vi "GetFileStringBmp.vi"(7 "Color Palette":T1[](array[typedef]), 8 "error in":errorcluster, 9 "Base64 Encoded":bool, 10 "Compress":bool, 11 "Image Reference In":T2) -> (0 "error out":errorcluster, 2 "FileString":string, 3 "Image Reference Out":T2)   [LabVIEW 2020, in "OpenLvVision_Image.lvlib" / "File.lvlib"]
doc: "Returns the entire image content encoded as a string representing an image file, suitable for saving or transferring over the network."
uses:
  File.lvlib
  Management/TypeDef/Image.ctl
  TypeDef/ColorPaletteValue.ctl
  Management/Management.lvlib
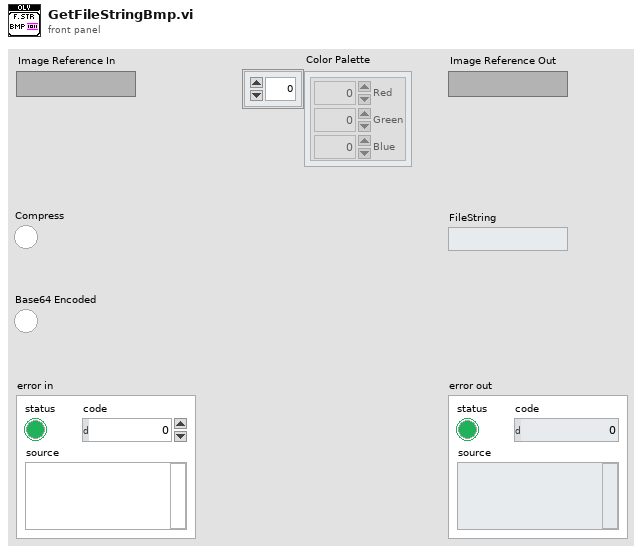
[diagram p1: front panel]
types:
  T1 = typedef "OpenLvVision_Image.lvlib/File.lvlib/ColorPaletteValue.ctl" = cluster{"Red":u8, "Green":u8, "Blue":u8}
  T2 = typedef "OpenLvVision_Image.lvlib/Management.lvlib/Image.ctl" = refnum<image>
  T3 = typedef "IMAQ Image.ctl" = refnum<image>
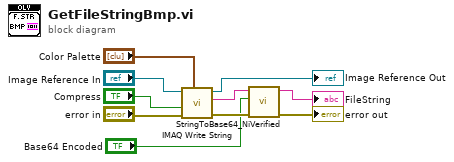
[diagram p0: block diagram]
diagram:
  n1 = call-poly "IMAQ Write String"("Color Palette"="Color Palette", "error in (no error)"="error in", "Compress? (N)"="Compress", "Image"="Image Reference In") -> ("error out"=w5:errorcluster, "File String Out"=w2:string, "Image Out (duplicate)"=→"Image Reference Out":T3)  [unwired: 5 in]
  n2 = call "StringToBase64_NiVerified.vi"("error in"=w5, "Encode"="Base64 Encoded", "RawString"=w2) -> ("error out"=→"error out":errorcluster, "EncodedString"=→"FileString":string)  [unwired: 7 in]
